vi "GetObjectClassType.vi"(3 "type string":i16[](array[numeric])) -> (0 "type":T1(ring), 1 "duplicate type string":i16[](array[numeric]))   [LabVIEW 2020, in "OpenG_Object.lvclass"]
doc: "Finds out if an object specified by the type string is a LabVIEW Object or a user specified object or neither."
uses:
  OpenG_Object.lvclass
panel:
  # "Please visit http://www.OpenG.org to learn about the\nOpen Source LabVIEW software movement.\n\nNOTICE -- YOU MUST LEAVE THIS NOTICE IN PLACE.  PER THE TERMS OF THE LICENSE BELOW, YOU MAY SUBLICENSE THIS SOFTWARE \nIN ANY WAY THAT DOES NOT CONFLICT WITH THIS LICENSE.\n\n### BSD License (http://www.opensource.org/licenses/bsd-license.php) Begin ###\n\nCopyright (c) 2007, Tomi Maila\nCopyright (c) 2007, Endevo AB\n\n\nAll rights reserved.\n\nRedistribution and use in source and binary forms, with or without modification, are permitted provided that the following conditions are met:\n\n    * Redistributions of source code must retain the above copyright notice, this list of conditions and the following disclaimer.\n    * Redistributions in binary form must reproduce the above copyright notice, this list of conditions and the following disclaimer in the \n       documentation and/or other materials provided with the distribution.\n    * Neither the name of Endevo AB nor the names of the contributors may be used to endorse or promote products derived\n       from this software without specific prior written permission.\n\nTHIS SOFTWARE IS PROVIDED BY THE COPYRIGHT HOLDERS AND CONTRIBUTORS \"AS IS\" AND ANY EXPRESS OR IMPLIED WARRANTIES, \nINCLUDING, BUT NOT LIMITED TO, THE IMPLIED WARRANTIES OF MERCHANTABILITY AND FITNESS FOR A PARTICULAR PURPOSE ARE \nDISCLAIMED. IN NO EVENT SHALL THE COPYRIGHT OWNER OR CONTRIBUTORS BE LIABLE FOR ANY DIRECT, INDIRECT, INCIDENTAL,\n SPECIAL, EXEMPLARY, OR CONSEQUENTIAL DAMAGES (INCLUDING, BUT NOT LIMITED TO, PROCUREMENT OF SUBSTITUTE GOODS OR \nSERVICES; LOSS OF USE, DATA, OR PROFITS; OR BUSINESS INTERRUPTION) HOWEVER CAUSED AND ON ANY THEORY OF LIABILITY, \nWHETHER IN CONTRACT, STRICT LIABILITY, OR TORT (INCLUDING NEGLIGENCE OR OTHERWISE) ARISING IN ANY WAY OUT OF THE USE \nOF THIS SOFTWARE, EVEN IF ADVISED OF THE POSSIBILITY OF SUCH DAMAGE.\n\n### BSD License End ###"
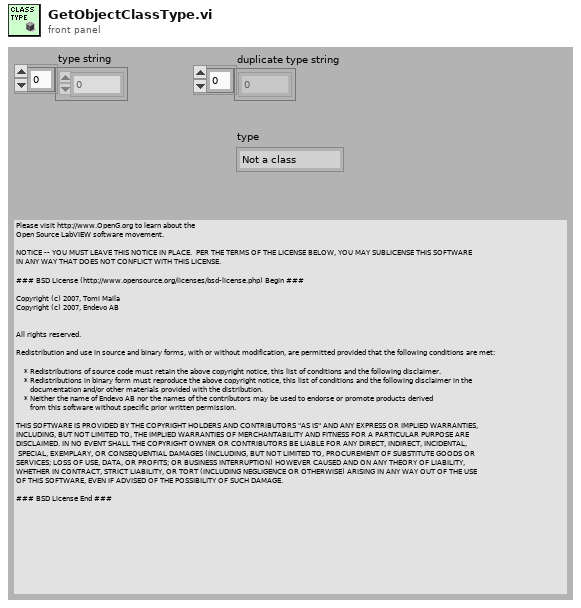
[diagram p1: front panel]
types:
  T1 = enum16{"Not a class", "LabVIEW Object", "Normal Class"}
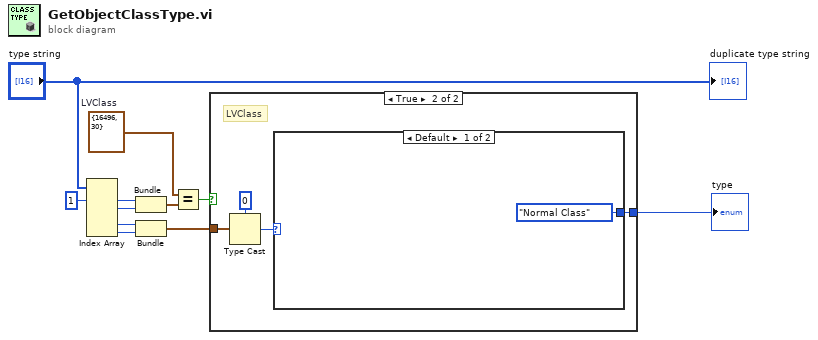
[diagram p0: block diagram]
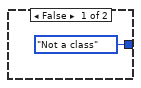
[diagram p2: hidden frame]
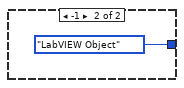
[diagram p3: hidden frame]
diagram:
  w4 = cluster{"Numeric":i16, "Numeric":i16} {"Numeric"=16496, "Numeric"=30}  # LVClass
  n1 = Index Array(array="type string", index #1=1 ("index")) -> (element #1=w8:i16, element #2=w9:i16, element #4=w7:i16, element #5=w6:i16)  [unwired: 4 in, 1 out]
  n2 = Bundle("Numeric"=w8, "Numeric"=w9) -> (w5:cluster{"Numeric":i16, "Numeric":i16})  [unwired: 1 in]
  n3 = Bundle("Numeric"=w7, "Numeric"=w6) -> (w2:cluster{"Numeric":i16, "Numeric":i16})  [unwired: 1 in]
  n4 = Equal?(x=w4, y=w5) -> (x = y?=w3:bool)
  n5 = case shown="True" w3 {
    tunnel: w2 -> [_ w16]
    tunnel: [T1."Not a class" ("type") w13] -> w1
    frame False {
    }
    frame True {
      # "LVClass"
      n6 = Type Cast(type=0, x=w16) -> (*(type *) &x=w15:i32)
      n7 = case shown="Default" w15 {
        tunnel: [T1."Normal Class" ("type") T1."LabVIEW Object" ("type")] -> w13
        frame Default {
        }
        frame -1 {
        }
      }
    }
  }
  "type" <- w1
  "duplicate type string" <- "type string"
